vi "Build_Status_String.vi"(1 "Alias Table":string[][](array[string]), 2 "Status Array":T1(array[cluster]), 3 "Event":cluster{string, string[], dbl[], dbl}) -> (0 "Status":string)   [LabVIEW 2011]
doc: "This VI uses the \"Event\" and \"Status Array\" parameters to find the appropriate \"Status\" for a given event. The \"Status\" is an arbitrarily formatted multi-line text block that is intended to give the growth sequence operator a general overview of the currently selected event. This could include information such as current flow rate or temperature."
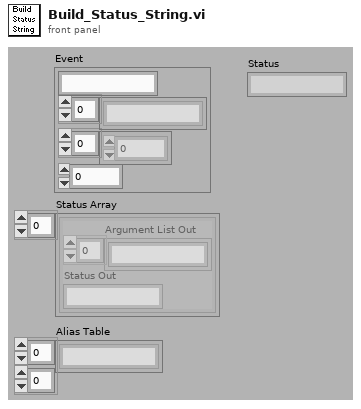
[diagram p1: front panel]
types:
  T1 = cluster{"Argument List Out":string[], "Status Out":string}[]
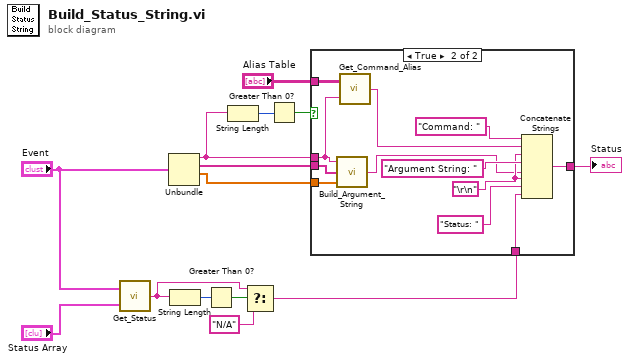
[diagram p0: block diagram]
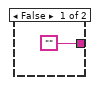
[diagram p2: hidden frame]
diagram:
  n1 = call "Get_Status.vi"("Status Array"="Status Array", "Event"="Event") -> ("Status"=w8:string)
  n2 = Unbundle("Event") -> (w2:string, w12:string[], w11:dbl[])  [unwired: 1 out]
  n3 = String Length(string=w8) -> (length=w10:i32)
  n4 = Greater Than 0?(x=w10) -> (x > 0?=w9:bool)
  n5 = String Length(string=w2) -> (length=w3:i32)
  n6 = Select(t=w8, s=w9, f="N/A") -> (s? t:f=w6:string)
  n7 = Greater Than 0?(x=w3) -> (x > 0?=w4:bool)
  n8 = case shown="True" w4 {
    tunnel: w12 -> [_ w27]
    tunnel: w11 -> [_ w26]
    tunnel: w2 -> [_ w17]
    tunnel: w6 -> [_ w20]
    tunnel: ["" w19] -> w5
    tunnel: "Alias Table" -> [_ w18]
    frame False {
    }
    frame True {
      w23 = "\r\n"
      n9 = call "Build_Argument_String.vi"("Flow Array"=w26, "Argument List"=w27, "Command"=w17) -> ("Argument String"=w21:string)
      n10 = call "Get_Command_Alias.vi"("Command"=w17, "Alias Table"=w18) -> ("Alias"=w16:string)
      n11 = Concatenate Strings("Command: " ("string"), w16, w23, "Argument String: " ("string"), w21, w23, "Status: " ("string"), w20) -> (w19:string)
    }
  }
  "Status" <- w5
